vi "Setpoints.vi"() -> ()   [LabVIEW 2014]
uses:
  <userlib>/Nanonis Prog Interface V5/Nanonis Prog Interface.lvlib
panel:
  in  "Get1 3":bool
  in  "Set1 3":bool
  in  "Current 3":dbl format="%#_6p"
  in  "Bias 3":dbl format="%#_6p"
  in  "Current 2":dbl format="%#_6p"
  in  "Bias 2":dbl format="%#_6p"
  in  "Get1 2":bool
  in  "Set1 2":bool
  in  "stop":bool
  in  "Get1":bool
  in  "Current":dbl format="%#_6p"
  in  "Bias":dbl format="%#_6p"
  in  "Set1":bool
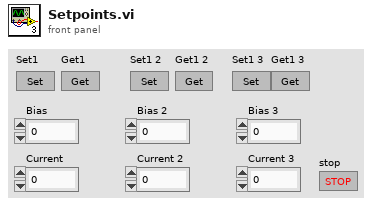
[diagram p1: front panel]
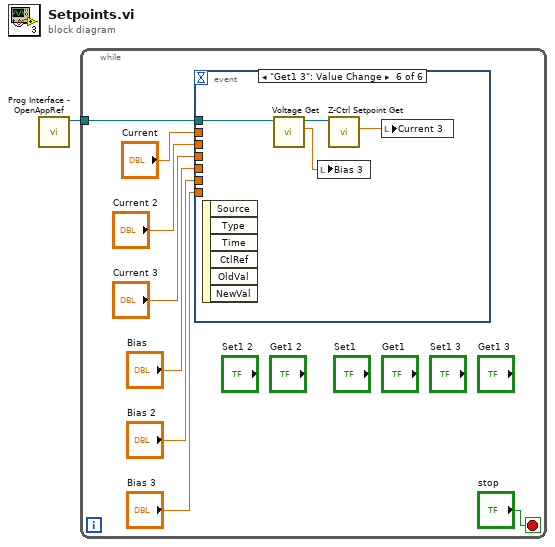
[diagram p0: block diagram]
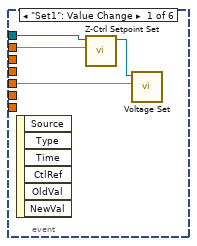
[diagram p2: hidden frame]
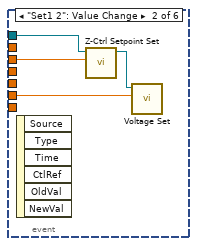
[diagram p3: hidden frame]
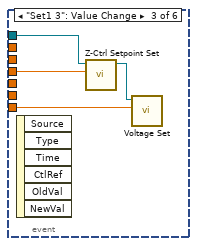
[diagram p4: hidden frame]
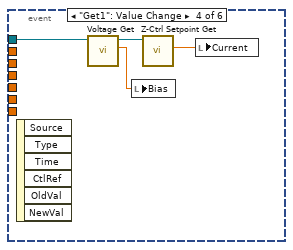
[diagram p5: hidden frame]
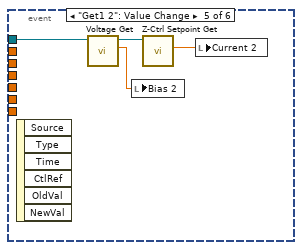
[diagram p6: hidden frame]
diagram:
  n1 = call <userlib>:"Prog Interface - OpenAppRef.vi"() -> ("Application reference"=w1:refnum<vi>)  [unwired: 6 in, 1 out]
  n2 = while {
    tunnel: w1 -> [w6]
    stop <- "stop" stop-if-true
    n3 = event shown="[5] \"Get1 3\": Value Change" {
      selector: _ -> [_ _ _ _ _ _]
      dyn-events: _ -> [_ _ _ _ _ _]
      timeout: _ -> [_ _ _ _ _ _]
      tunnel: "Current" -> [w13 _ _ _ _ _]
      tunnel: "Bias" -> [w12 _ _ _ _ _]
      tunnel: w6 -> [w10 w16 w20 w25 w29 w33]
      tunnel: "Current 2" -> [_ w15 _ _ _ _]
      tunnel: "Bias 2" -> [_ w14 _ _ _ _]
      tunnel: "Current 3" -> [_ _ w19 _ _ _]
      tunnel: "Bias 3" -> [_ _ w18 _ _ _]
      event "Set1": Value Change {
        n4 = event-data() -> ()  [unwired: 1 in, 6 out]
        n5 = call <userlib>:"Z-Ctrl Setpoint Set.vi"("Z Controller setpoint"=w13, "Application ref in"=w10) -> ("Application ref out"=w11:refnum<vi>)  [unwired: 8 in, 1 out]
        n6 = call <userlib>:"Voltage Set.vi"("Bias (V)"=w12, "Application ref in"=w11) -> ()  [unwired: 8 in, 2 out]
      }
      event "Set1 2": Value Change {
        n7 = event-data() -> ()  [unwired: 1 in, 6 out]
        n8 = call <userlib>:"Z-Ctrl Setpoint Set.vi"("Z Controller setpoint"=w15, "Application ref in"=w16) -> ("Application ref out"=w17:refnum<vi>)  [unwired: 8 in, 1 out]
        n9 = call <userlib>:"Voltage Set.vi"("Bias (V)"=w14, "Application ref in"=w17) -> ()  [unwired: 8 in, 2 out]
      }
      event "Set1 3": Value Change {
        n10 = event-data() -> ()  [unwired: 1 in, 6 out]
        n11 = call <userlib>:"Z-Ctrl Setpoint Set.vi"("Z Controller setpoint"=w19, "Application ref in"=w20) -> ("Application ref out"=w21:refnum<vi>)  [unwired: 8 in, 1 out]
        n12 = call <userlib>:"Voltage Set.vi"("Bias (V)"=w18, "Application ref in"=w21) -> ()  [unwired: 8 in, 2 out]
      }
      event "Get1": Value Change {
        n13 = event-data() -> ()  [unwired: 1 in, 6 out]
        n14 = call <userlib>:"Voltage Get.vi"("Application ref in"=w25) -> ("Bias (V)"=w23:sgl, "Application ref out"=w24:refnum<vi>)  [unwired: 8 in, 1 out]
        n15 = local write "Bias"(w23) -> ()
        n16 = call <userlib>:"Z-Ctrl Setpoint Get.vi"("Application ref in"=w24) -> ("Z Controller setpoint"=w22:sgl)  [unwired: 7 in, 2 out]
        n17 = local write "Current"(w22) -> ()
      }
      event "Get1 2": Value Change {
        n18 = event-data() -> ()  [unwired: 1 in, 6 out]
        n19 = call <userlib>:"Voltage Get.vi"("Application ref in"=w29) -> ("Bias (V)"=w27:sgl, "Application ref out"=w28:refnum<vi>)  [unwired: 8 in, 1 out]
        n20 = local write "Bias 2"(w27) -> ()
        n21 = call <userlib>:"Z-Ctrl Setpoint Get.vi"("Application ref in"=w28) -> ("Z Controller setpoint"=w26:sgl)  [unwired: 7 in, 2 out]
        n22 = local write "Current 2"(w26) -> ()
      }
      event "Get1 3": Value Change {
        n23 = event-data() -> ()  [unwired: 1 in, 6 out]
        n24 = call <userlib>:"Voltage Get.vi"("Application ref in"=w33) -> ("Bias (V)"=w31:sgl, "Application ref out"=w32:refnum<vi>)  [unwired: 8 in, 1 out]
        n25 = local write "Bias 3"(w31) -> ()
        n26 = call <userlib>:"Z-Ctrl Setpoint Get.vi"("Application ref in"=w32) -> ("Z Controller setpoint"=w30:sgl)  [unwired: 7 in, 2 out]
        n27 = local write "Current 3"(w30) -> ()
      }
    }
  }
